vi "mainActivity_元素入队列.vi"(8 "error in (no error)":errorcluster caption="错误输入（无错误）", 11 "元素":cluster{"消息":string, "数据":variant}) -> (0 "error out":errorcluster caption="错误输出")   [LabVIEW 2014]
doc: "该模板用于创建子VI。"
uses:
  R/manifest.vi
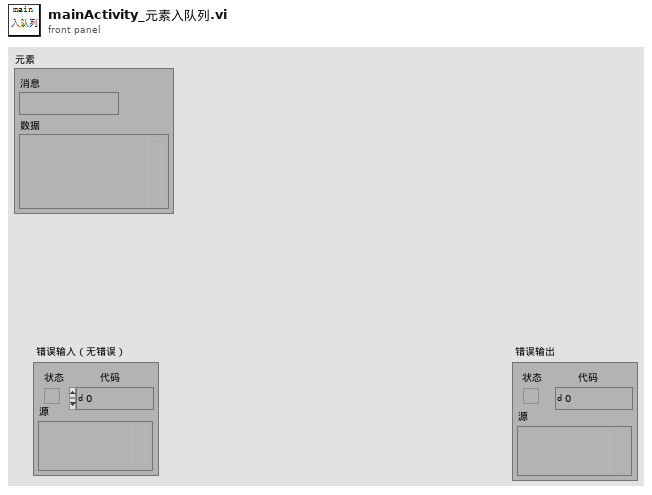
[diagram p1: front panel]
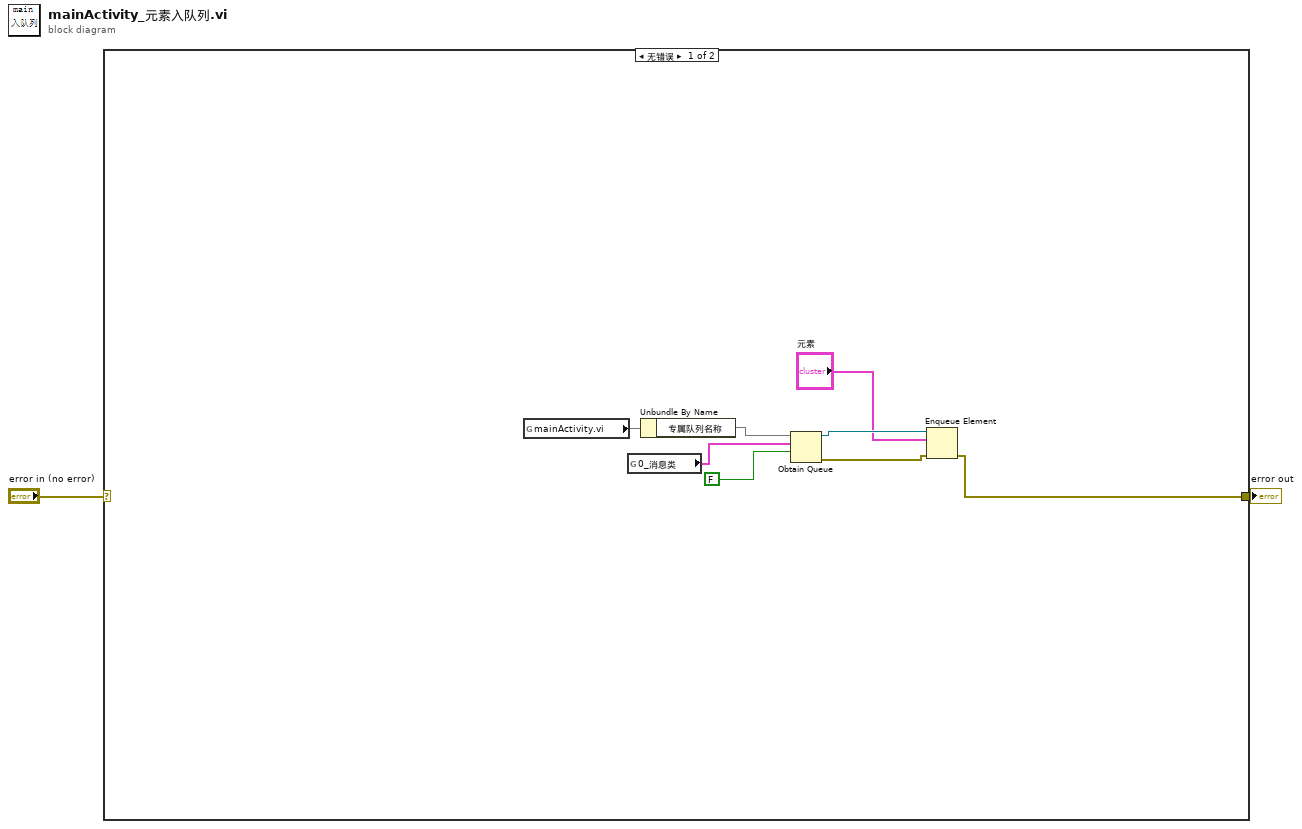
[diagram p0: block diagram]
diagram:
  n1 = case shown="无错误" "error in (no error)" {
    selector: "error in (no error)" -> [_ w11]
    tunnel: [w3 w11] -> w1
    frame No Error {
      n2 = global read "manifest.vi" "mainActivity.vi"() -> (w10)
      n3 = global read "类信息.vi" "0_消息类"() -> (w7:cluster{"消息":string, "数据":variant})
      n4 = Unbundle By Name(w10) -> ("专属队列名称"=w9)
      n5 = Obtain Queue(name (unnamed)=w9, element data type=w7, create if not found? (T)=FALSE ("如未找到是否创建？(T)")) -> (queue out=w5:refnum<queue>, error out=w6:errorcluster)  [unwired: 2 in, 1 out]
      n6 = Enqueue Element(queue=w5, element="元素", error in (no error)=w6) -> (error out=w3:errorcluster)  [unwired: 1 in, 2 out]
    }
    frame Error {
    }
  }
  "error out" <- w1
